vi "ZC_pandian.vi"(0 "name":string, 1 "LabVIEW Web Service Request":refnum<class "Web Request.lvclass"> caption="LabVIEW Web服务请求", 2 "beizhu":string, 3 "number":string, 5 "jzriqi":string, 7 "status":string, 9 "shchriqi":string, 11 "action":string, 12 "key":string, 13 "id":string) -> (4 "error":errorcluster)   [LabVIEW 2017]
uses:
  <vilib>/wsapi/Web Request.lvclass
panel:
  out "error 2":errorcluster caption="error"
  out "postdata":string caption="post数据"
  out "error out":errorcluster caption="错误输出"
  # "Web服务请求输入接线端用于调用“Web服务”选板的VI。除非不需要访问该选板，否则不要在连线板上删除这个输入接线端。"
  # "添加至连线板的每一个其他输入控件，在URL中对应于一个输入。如需在接线端模式输出（默认设置）下包含显示控件，则该显示控件必须与连线板相连。"
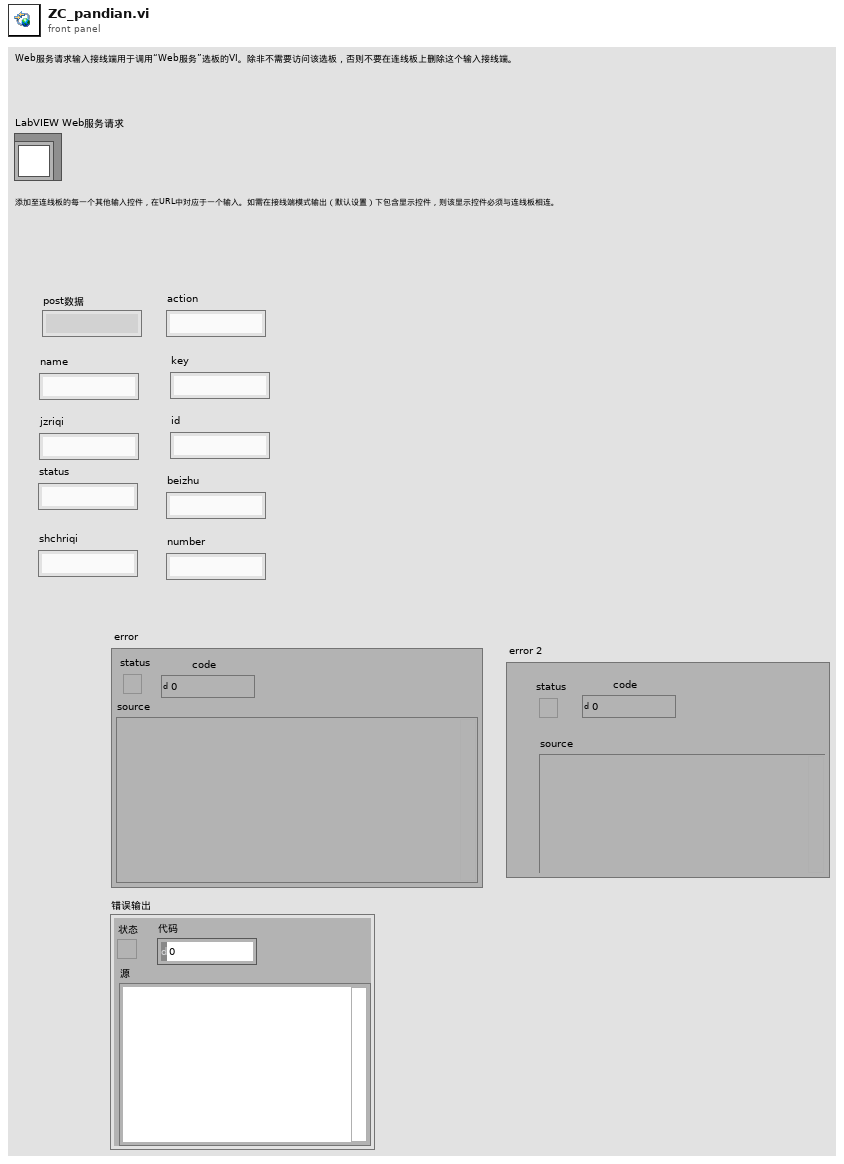
[diagram p1: front panel]
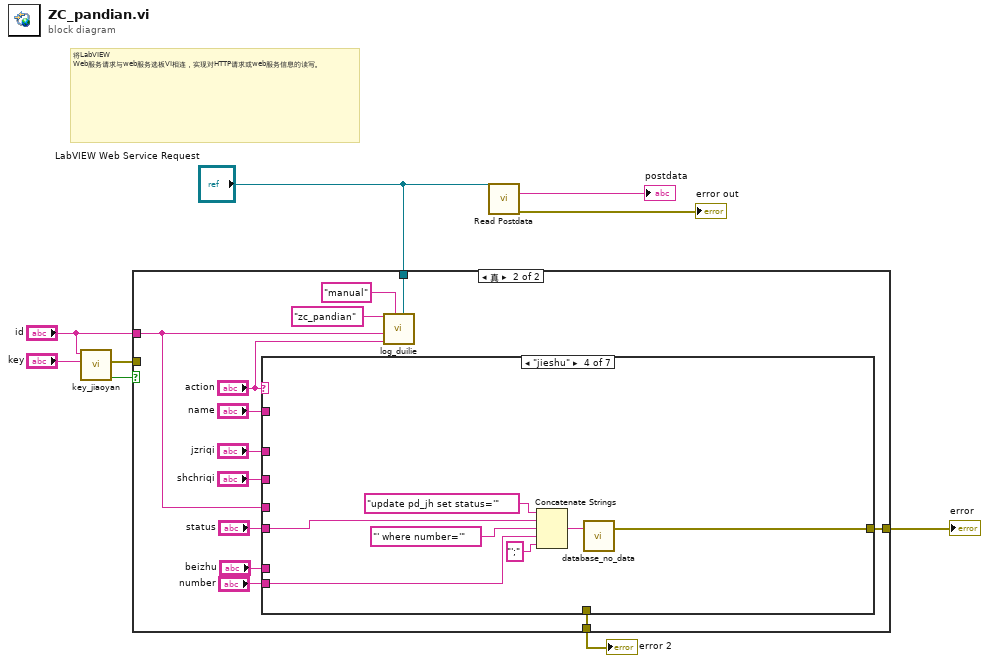
[diagram p0: block diagram]
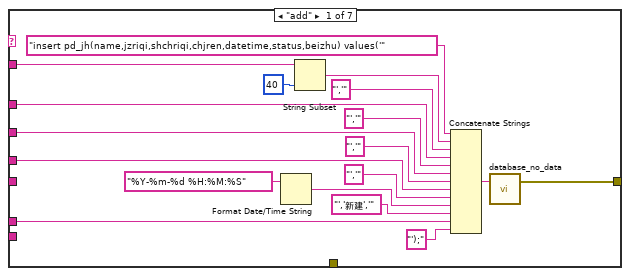
[diagram p3: hidden frame]
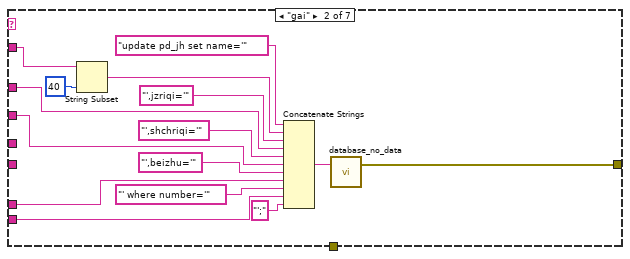
[diagram p4: hidden frame]
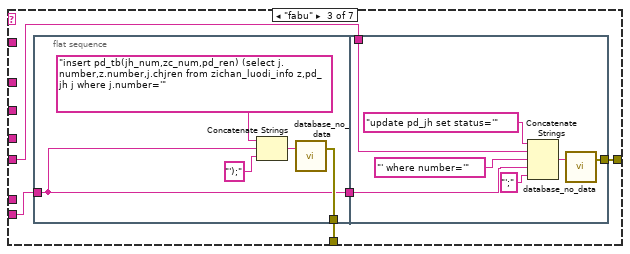
[diagram p5: hidden frame]
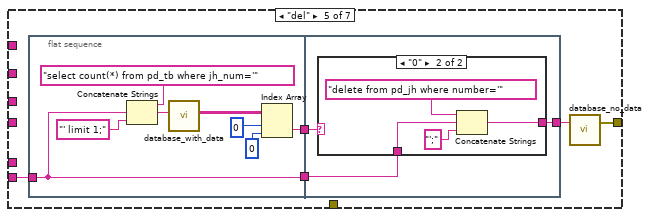
[diagram p6: hidden frame]
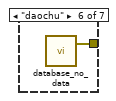
[diagram p8: hidden frame]
diagram:
  # "将LabVIEW Web服务请求与web服务选板VI相连，实现对HTTP请求或web服务信息的读写。"
  n1 = call "key_jiaoyan.vi"("key_client"="key", "gonghao"="id") -> ("jy"=w4:bool, "error"=w3:errorcluster)  [unwired: 8 in]
  n2 = case shown="真" w4 {
    tunnel: [w10 w18] -> w8
    tunnel: "LabVIEW Web Service Request" -> [_ w15]
    tunnel: "id" -> [_ w13]
    tunnel: w3 -> [w10 _]
    tunnel: [_ w11] -> w1
    frame False {
    }
    frame True {
      n3 = case shown="\"jieshu\"" "action" {
        tunnel: [w33 w49 w61 w78 w81 w101 _] -> w18
        tunnel: "shchriqi" -> [w30 w46 _ _ _ _ _]
        tunnel: "beizhu" -> [w24 w45 _ _ _ _ _]
        tunnel: w13 -> [w29 _ _ _ _ _ _]
        tunnel: "jzriqi" -> [w31 w47 _ _ _ _ _]
        tunnel: "name" -> [w32 w48 _ _ _ _ _]
        tunnel: "number" -> [_ w43 w58 w76 w82 _ _]
        tunnel: "status" -> [_ _ w60 w74 _ _ _]
        tunnel: [_ _ w59 _ _ _ _] -> w11
        frame "add" {
          n4 = Format Date/Time String(time format string (%c)="%Y-%m-%d %H:%M:%S" ("时间格式字符串(%c)")) -> (date/time string=w27:string)  [unwired: 2 in]
          n5 = String Subset(string=w32, length (rest)=40 ("长度（剩余）")) -> (substring=w38:string)  [unwired: 1 in]
          n6 = Concatenate Strings("insert pd_jh(name,jzriqi,shchriqi,chjren,datetime,status,beizhu) values('" ("格式字符串"), w38, "','" ("字符串"), w31, "','" ("字符串"), w30, "','" ("字符串"), w29, "','" ("字符串"), w27, "','新建','" ("字符串"), w24, "');" ("字符串")) -> (w34:string)
          n7 = call "database_no_data.vi"("input"=w34) -> ("error"=w33:errorcluster)  [unwired: 2 in]
        }
        frame "gai" {
          n8 = String Subset(string=w48, length (rest)=40 ("长度（剩余）")) -> (substring=w53:string)  [unwired: 1 in]
          n9 = Concatenate Strings("update pd_jh set name='" ("格式字符串"), w53, "',jzriqi='" ("字符串"), w47, "',shchriqi='" ("字符串"), w46, "',beizhu='" ("字符串"), w45, "' where number='" ("字符串"), w43, "';" ("字符串")) -> (w50:string)
          n10 = call "database_no_data.vi"("input"=w50) -> ("error"=w49:errorcluster)  [unwired: 2 in]
        }
        frame "fabu" {
          n11 = flat-sequence {
            tunnel: [w63] -> w59
            tunnel: w58 -> [w62]
            tunnel: [w62] -> w57
            tunnel: [w71] -> w61
            tunnel: w60 -> [w68]
            tunnel: w57 -> [w67]
            frame #0 {
              n12 = Concatenate Strings("insert pd_tb(jh_num,zc_num,pd_ren) (select j.number,z.number,j.chjren from zichan_luodi_info z,pd_jh j where j.number='" ("格式字符串"), w62, "');" ("字符串")) -> (w66:string)
              n13 = call "database_no_data.vi"("input"=w66) -> ("error"=w63:errorcluster)  [unwired: 2 in]
            }
            frame #1 {
              n14 = Concatenate Strings("update pd_jh set status='" ("格式字符串"), w68, "' where number='" ("字符串"), w67, "';" ("字符串")) -> (w72:string)
              n15 = call "database_no_data.vi"("input"=w72) -> ("error"=w71:errorcluster)  [unwired: 2 in]
            }
          }
        }
        frame "jieshu" {
          n16 = Concatenate Strings("update pd_jh set status='" ("格式字符串"), w74, "' where number='" ("字符串"), w76, "';" ("字符串")) -> (w79:string)
          n17 = call "database_no_data.vi"("input"=w79) -> ("error"=w78:errorcluster)  [unwired: 2 in]
        }
        frame "del" {
          n18 = flat-sequence {
            tunnel: w82 -> [w91]
            tunnel: [w91] -> w85
            tunnel: [w86] -> w84
            tunnel: [w96] -> w83
            tunnel: w85 -> [w95]
            tunnel: w84 -> [w94]
            frame #0 {
              n19 = Concatenate Strings("select count(*) from pd_tb where jh_num='" ("格式字符串"), w91, "' limit 1;" ("字符串")) -> (w90:string)
              n20 = call "database_with_data.vi"("input"=w90) -> ("Data"=w87:string[][])  [unwired: 9 in, 1 out]
              n21 = Index Array(array=w87, index (row)=0 ("索引 (行)"), index (col)=0 ("禁用的索引 (列)")) -> (element=w86:string)
            }
            frame #1 {
              n22 = case shown="\"0\"" w94 {
                tunnel: [_ w98] -> w96
                tunnel: w95 -> [_ w97]
                frame "假", Default {
                }
                frame "0" {
                  n23 = Concatenate Strings("delete from pd_jh where number='" ("格式字符串"), w97, "';" ("字符串")) -> (w98:string)
                }
              }
            }
          }
          n24 = call "database_no_data.vi"("input"=w83) -> ("error"=w81:errorcluster)  [unwired: 2 in]
        }
        frame "daochu" {
          n25 = call "database_no_data.vi"() -> ("error"=w101:errorcluster)  [unwired: 3 in]
        }
        frame Default {
        }
      }
      n26 = call "log_duilie.vi"("LabVIEW Web Service Request"=w15, "type"="manual", "action"="action", "user"=w13, "yw"="zc_pandian") -> ()  [unwired: 7 in]
    }
  }
  "error" <- w8
  "error 2" <- w1
  n27 = call <vilib>:"Read Postdata.vi"("LabVIEW Web Service Request"="LabVIEW Web Service Request") -> ("postdata"=→"postdata":string, "error out"=→"error out":errorcluster)  [unwired: 12 in, 1 out]
